vi "Scanner_Testing_1.vi"() -> ()   [LabVIEW 2017]
panel:
  in  "mode (standard)":T1(ring)
  in  "address":string="192.168.0.71"
  in  "remote port or service name":u16=8080
  out "error out":errorcluster
  out "data out":string
  in  "stop":bool
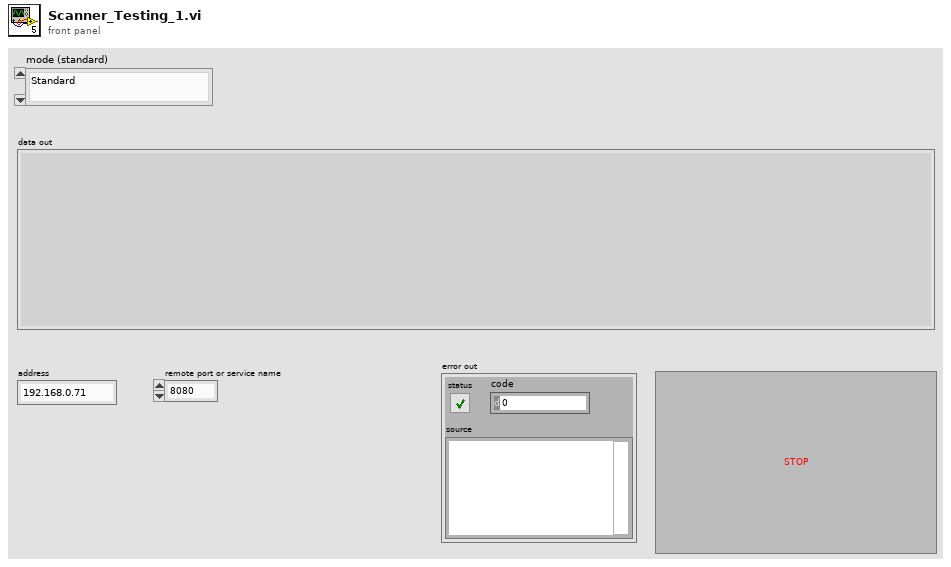
[diagram p1: front panel]
types:
  T1 = enum16{"Standard", "Buffered", "CRLF", "Immediate"}
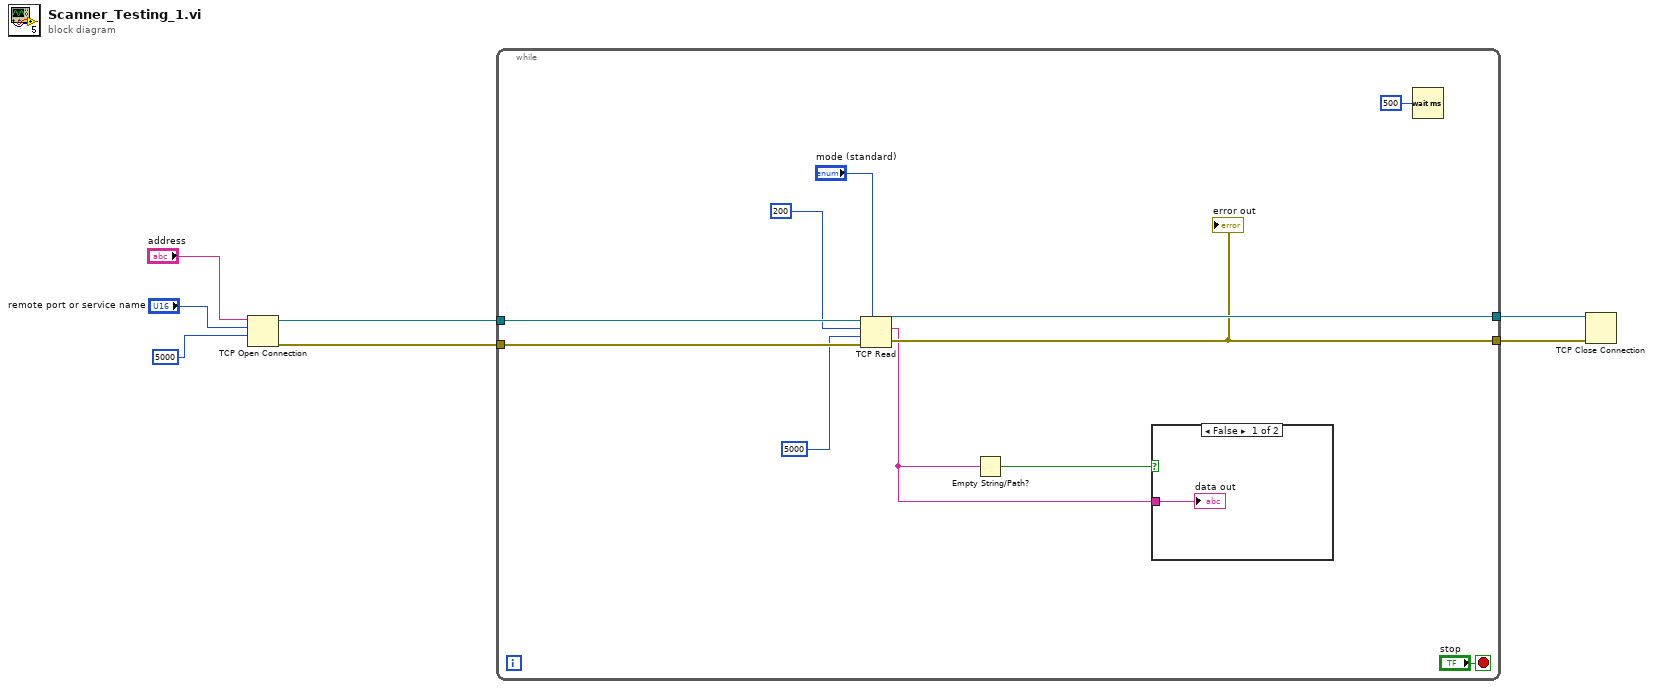
[diagram p0: block diagram]
diagram:
  n1 = TCP Open Connection(address="address", remote port or service name="remote port or service name", timeout ms (60000)=5000) -> (connection ID=w7:refnum<k5>, error out=w6:errorcluster)  [unwired: 2 in]
  n2 = while {
    tunnel: w7 -> [w16]
    tunnel: w6 -> [w15]
    tunnel: [w14] -> w5
    tunnel: [w13] -> w4
    stop <- "stop" stop-if-true
    n3 = TCP Read(connection ID=w16, bytes to read=200, error in (no error)=w15, 7:"mode (standard)", 9:5000 ("timeout ms (25000)")) -> (connection ID out=w14:refnum<k5>, data out=w10:string, error out=w13:errorcluster)
    "error out" <- w13
    n4 = Empty String/Path?(string/path=w10) -> (empty?=w9:bool)
    n5 = case shown="False" w9 {
      tunnel: w10 -> [w19 _]
      frame False {
        "data out" <- w19
      }
      frame True {
      }
    }
    n6 = Wait (ms)(milliseconds to wait=u32 500) -> ()  [unwired: 1 out]
  }
  n7 = TCP Close Connection(connection ID=w5, error in (no error)=w4) -> ()  [unwired: 1 in, 2 out]
